vi "PG Path to Plot Label From Cursor.vi"(8 "error in (no error)":errorcluster, 9 "Time Stamp":timestamp, 10 "PG Path":string, 11 "Database Viewer":refnum<class "Database Viewer.lvclass">) -> (0 "error out":errorcluster, 2 "Plot Label":string, 3 "Database Viewer":refnum<class "Database Viewer.lvclass">)   [LabVIEW 2019, in "Database Viewer.lvclass"]
uses:
  Database Viewer.lvclass
  <userlib>/LevyLab/LV-Data/LV-Data.PG/API/Read Variable (string).vi
  <userlib>/LevyLab/LV-Data/LV-Data.PG/LV-Data.PGSQL.lvclass
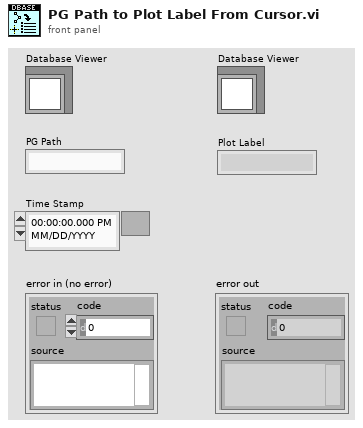
[diagram p1: front panel]
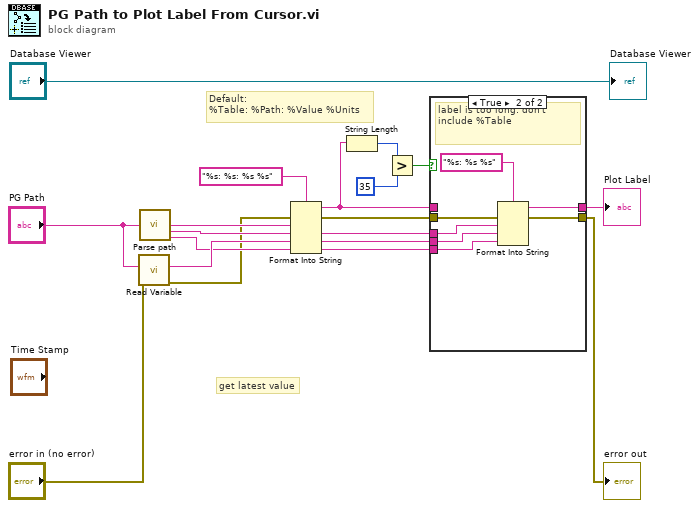
[diagram p0: block diagram]
diagram:
  # "get latest value"
  # "Default:\n%Table: %Path: %Value %Units"
  n1 = call-poly <userlib>:"Read Variable.vi"("error in (no error)"="error in (no error)", "PG path"="PG Path") -> ("error out"=w4:errorcluster, "Value"=w7:string)  [unwired: 4 in, 4 out]
  n2 = call <userlib>:"Parse path.vi"("PG Path"="PG Path") -> ("Table name"=w9:string, "Column name"=w8:string, "Column units"=w6:string)  [unwired: 10 in, 2 out]
  n3 = Format Into String(format string="%s: %s: %s %s", error in=w4, w9, w8, w7, w6) -> (resulting string=w2:string, error out=w5:errorcluster)  [unwired: 1 in]
  n4 = String Length(string=w2) -> (length=w14:i32)
  n5 = Greater?(x=w14, y=35) -> (0:w13:bool)
  n6 = case shown="True" w13 {
    tunnel: [w18 w21] -> w12
    tunnel: w2 -> [w18 _]
    tunnel: w8 -> [_ w24]
    tunnel: w7 -> [_ w23]
    tunnel: w6 -> [_ w22]
    tunnel: w5 -> [w17 w20]
    tunnel: [w17 w19] -> w3
    frame False {
    }
    frame True {
      # "label is too long: don't include %Table"
      n7 = Format Into String(format string="%s: %s %s", error in=w20, w24, w23, w22) -> (resulting string=w21:string, error out=w19:errorcluster)  [unwired: 1 in]
    }
  }
  "Plot Label" <- w12
  "error out" <- w3
  "Database Viewer" <- "Database Viewer"
